vi "2_2_PatchCore_Inference(Camera).vi"() -> ()   [LabVIEW 2020]
uses:
  <vilib>/Ngene/DeepLTK Anomaly Detection Addon/DeepLTK_Anomaly_Detection_Addon/API/Controls/NN_Paths.ctl
  <vilib>/Ngene/Deep Learning Toolkit/Toolkit/NN_Data/API/NN_Dims(C,H,W).ctl
  <vilib>/Ngene/Deep Learning Toolkit/Toolkit/NN_Network/Controls/NN_Device.ctl
  subVIs/Visualizer/Controls/Display_Options.ctl
  subVIs/Visualizer/Controls/ROI_Display_Options.ctl
  subVIs/Visualizer/Controls/Heatmap_Display_Options.ctl
  subVIs/Visualizer/Controls/ColorMap.ctl
  <vilib>/Ngene/DeepLTK Anomaly Detection Addon/DeepLTK_Anomaly_Detection_Addon/API/Controls/MinMax.ctl
  subVIs/Camera/Controls/Camera_Settings.ctl
  <vilib>/vision/driver/IMAQdx.llb/IMAQdx Camera Control Mode.ctl
  <vilib>/Ngene/DeepLTK Anomaly Detection Addon/DeepLTK_Anomaly_Detection_Addon/API/Controls/NNPC_Setup.ctl
  <vilib>/Ngene/DeepLTK Anomaly Detection Addon/DeepLTK_Anomaly_Detection_Addon/API/Controls/Feature_Scorer_Params.ctl
  <vilib>/Ngene/DeepLTK Anomaly Detection Addon/DeepLTK_Anomaly_Detection_Addon/API/Controls/Gaussian_Blur.ctl
  <vilib>/vision/driver/IMAQdx.llb/IMAQdx Buffer Number Mode.ctl
  <vilib>/Ngene/DeepLTK Anomaly Detection Addon/DeepLTK_Anomaly_Detection_Addon/API/NNPC_Predict/NNPC_Predict(Single).vi
  <vilib>/Ngene/DeepLTK Anomaly Detection Addon/DeepLTK_Anomaly_Detection_Addon/DeepLTK_Anomaly_Detection_Addon.lvlib
  <vilib>/ptbypt/NI_PtbyPt.lvlib
  <vilib>/vision/driver/NI_Vision_Acquisition_Software.lvlib
  <vilib>/Ngene/Deep Learning Toolkit/Toolkit/Deep_Learning_Toolkit_by_Ngene.lvlib
  <vilib>/Ngene/CuLab - GPU Accelerated Toolkit/Toolkit/CuLab.lvlib
panel:
  in  "Tab Control":enum32{"CFG", "Demo"}(tab)
  in  "Center_Crop_Size":i32=700
  in  "Device":T1=enum."GPU"
  in  "Trained_Model_Paths":T2={"CFG"=path "D:/working/NI_Connect_PCB/NNPC_PCB5__25_04_11__16_58_48/NNPC_PCB5.cfg", "BIN"=path "D:/working/NI_Connect_PCB/NNPC_PCB5__25_04_11__16_58_48/NNPC_PCB5.bin"}
  in  "Display_Options":T3={"ROI_Options"={"Color"=16711713, "Width"=4, "Drawing Mode"=enum."Frame"}, "Heatmap_Options"={"ColorMap"=enum."Jet", "Alpha"=0.4, "Heatmap Range"={"Min"=38.0, "Max"=-1.0}}, "Has GT?"=FALSE} {"Heatmap_Options"."Heatmap Range"."Min" format="%#_5g"}
  in  "Camera":refnum<k21>="cam3" caption="IMAQdx Session"
  in  "Rel Margin":sgl=0.02
  in  "Camera_Settings":T8={"Camera_Resolution"=39, "Focus"=20, "Exposure"=5, "Gain"=0, "WhiteB."=3000} {"WhiteB." min=2800 max=6500 step=1; "Gain" max=255 step=1; "Exposure" min=0 max=6 step=1; "Focus" step=17}
  out "Loop Time":dbl=0.04018187299996498 format="%.2ps"
  out "Preproc. Time":dbl=0.002760252000152832 format="%.2ps"
  in  "Image_Thrshld":sgl=-1.0 format="%_5g"
  out "Pixel_Score(Max)":sgl=85.97979
  out "Img_Score":sgl=89.875435
  in  "Pixel_Thrshld":sgl=56.0 format="%_5g"
  out "Dims_In":T9={"C"=3, "H"=448, "W"=448}
  in  "Stop":bool
  out "Inference Time":dbl=0.012982828999520279 format="%.2ps"
  out "Prediction":bool=TRUE
  out "Device 2":string="NVIDIA GeForce RTX 2080 Ti"
  out "FPS":dbl=0.012982828999520279 format="%.2ps"
  out "Anomaly Detection Results":T10(plugin-control)
  # "Unsupervised \nVisual Anomaly Detection"
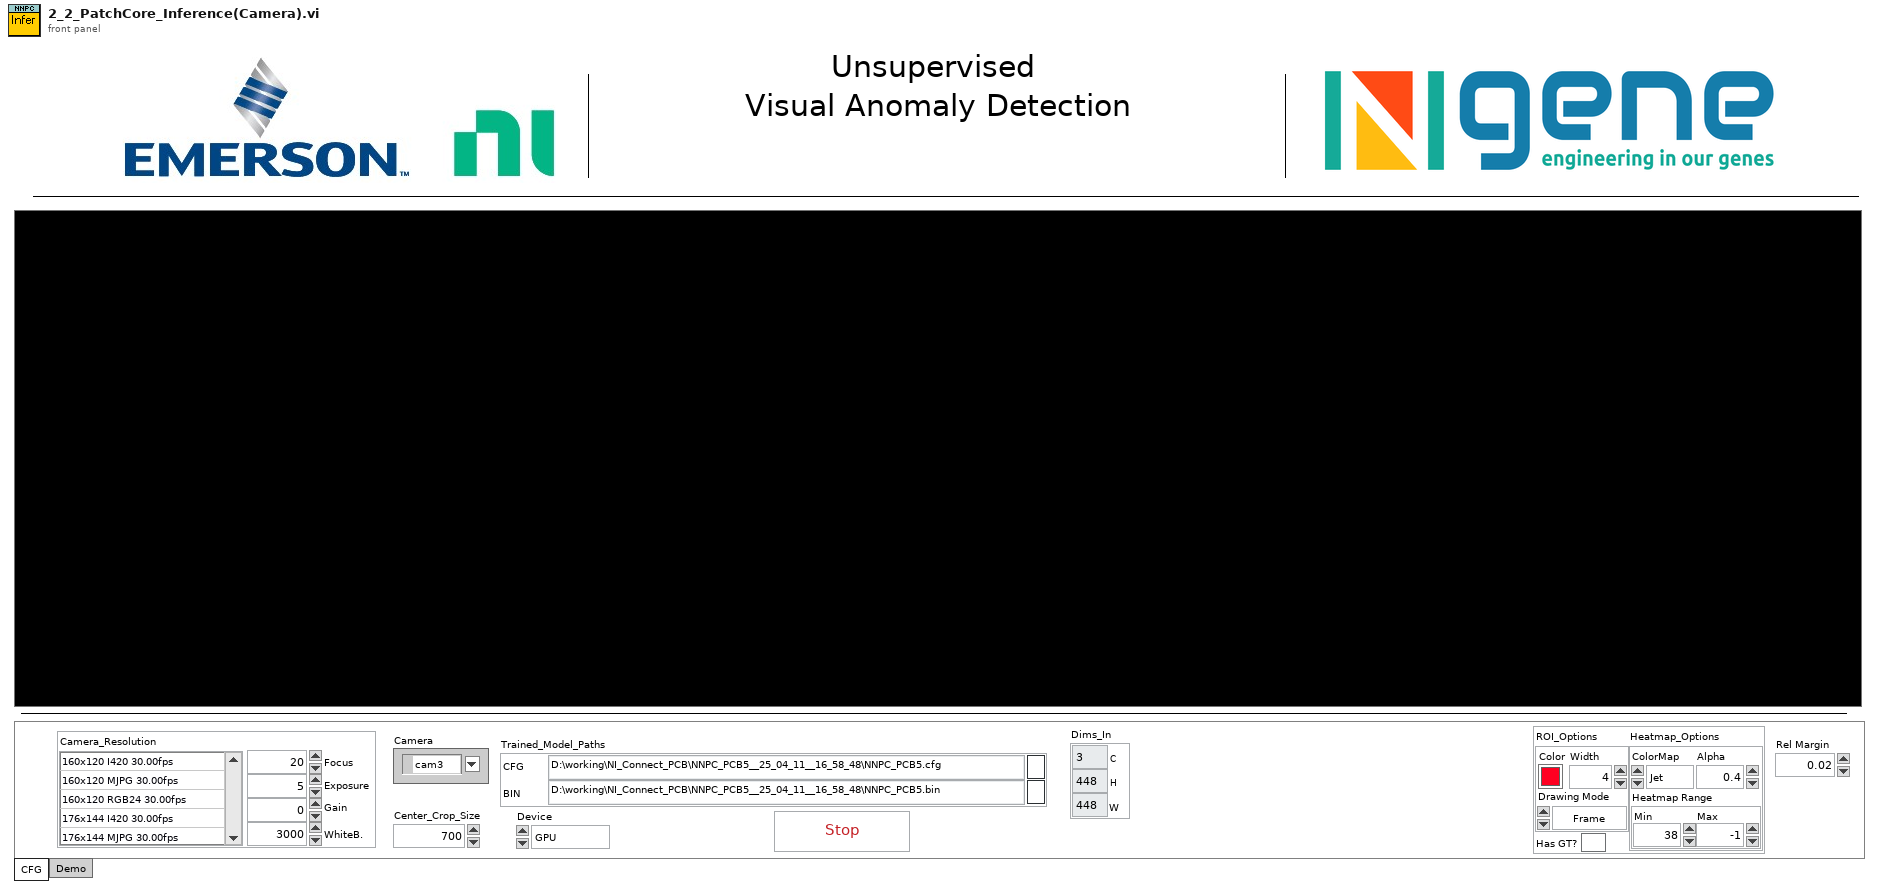
[diagram p1: front panel]
types:
  T1 = typedef "Deep_Learning_Toolkit_by_Ngene.lvlib/NN_Device.ctl" = enum16{"CPU", "GPU"}
  T2 = typedef "DeepLTK_Anomaly_Detection_Addon.lvlib/NN_Paths.ctl" = cluster{"CFG":path, "BIN":path}
  T3 = typedef "Display_Options.ctl" = cluster{"ROI_Options":T4, "Heatmap_Options":T5, "Has GT?":bool}
  T4 = typedef "ROI_Display_Options.ctl" = cluster{"Color":u32, "Width":u32, "Drawing Mode":enum16{"Frame", "Fill"}}
  T5 = typedef "Heatmap_Display_Options.ctl" = cluster{"ColorMap":T6, "Alpha":sgl, "Heatmap Range":T7}
  T6 = typedef "ColorMap.ctl" = enum16{"Jet", "Perula", "Inferno", "Plasma", "Viridis"}
  T7 = typedef "DeepLTK_Anomaly_Detection_Addon.lvlib/MinMax.ctl" = cluster{"Min":sgl, "Max":sgl}
  T8 = typedef "Camera_Settings.ctl" = cluster{"Camera_Resolution":i32, "Focus":u8, "Exposure":i32, "Gain":u32, "WhiteB.":i32}
  T9 = typedef "Deep_Learning_Toolkit_by_Ngene.lvlib/NN_Dims(C,H,W).ctl" = cluster{"C":i32, "H":i32, "W":i32}
  T10 = typedef "IMAQ Image.ctl" = refnum<image>
  T11 = typedef "NI_Vision_Acquisition_Software.lvlib/IMAQdx Camera Control Mode.ctl" = enum32{"Controller", "Listener"}
  T12 = typedef "Image Type" = u32
  T13 = typedef "DeepLTK_Anomaly_Detection_Addon.lvlib/NNPC_Setup.ctl" = cluster{"Input_Dims":T9, "mBatch":i32, "Device":T1, "GPU Id":i32}
  T14 = typedef "IMAQdx.ctl" = refnum<k21>
  T15 = typedef "DeepLTK_Anomaly_Detection_Addon.lvlib/NNPC_Evaluation_Results.ctl" = cluster{"Threshold(Image)":sgl, "Threshold(Pixel)":sgl, "Pixel_Range":cluster{"Min":sgl, "Max":sgl}}
  T16 = typedef "DeepLTK_Anomaly_Detection_Addon.lvlib/NNPC_PreProcessing_Options.ctl" = cluster{"DS_Name":string, "Input_Dims":T9, "Center Crop Size":i32, "Interpolation Type":u32, "Multi-Stage_DownSample?":bool, "Dataset_Stats":T17}
  T17 = typedef "DeepLTK_Anomaly_Detection_Addon.lvlib/NNPC_DS_Stats.ctl" = cluster{"means":T18, "stds":T18}
  T18 = typedef "DeepLTK_Anomaly_Detection_Addon.lvlib/Image_Stats_RGB.ctl" = cluster{"R":sgl, "G":sgl, "B":sgl}
  T19 = typedef "DeepLTK_Anomaly_Detection_Addon.lvlib/NNPC_Instance.ctl" = cluster{"NN":T20, "MemBank_Data":T35, "Name":string}
  T20 = typedef "Deep_Learning_Toolkit_by_Ngene.lvlib/NN.ctl" = cluster{"Name":string, "No of Layers":i32, "mBatch":i32, "Layers":T21[], "Dimty":T22, "Dims_In":T9, "Dims_Out":T9, "Working_Dir":path, "Train?":bool, "Train_Params":T23, "LR_Update_Policy":T26, "Session Data":T28, "Ground_truth":T29, "NNg_hdls":T30, "NN_Device":T1, "GPU Id":i32, "Labels":string[], "Receptive Field":T31[], "Loss_Type":T32, "Loss_Cfg_Prms":variant, "NNG_WS":T33}
  T21 = typedef "Deep_Learning_Toolkit_by_Ngene.lvlib/NN_Layer_ref.ctl" = refnum<data-value>
  T22 = typedef "Deep_Learning_Toolkit_by_Ngene.lvlib/NN_In_Out_Dim-ty.ctl" = enum8{"In1D_Out1D", "In3D_Out1D", "In3D_Out3D", "In3D_OutBBox"}
  T23 = typedef "Deep_Learning_Toolkit_by_Ngene.lvlib/NN_Train_Params.ctl" = cluster{"Optimizer":T24, "Beta_1":sgl, "Beta_2":sgl, "Weight Decay(L1)":sgl, "Weight Decay(L2)":sgl, "Data_Sampling":T25}
  T24 = typedef "Deep_Learning_Toolkit_by_Ngene.lvlib/NN_Train_Optimizer.ctl" = enum16{"SGD", "Adam", "Adagrad", "Adadelta", "RMSProp", "Nesterov"}
  T25 = typedef "Deep_Learning_Toolkit_by_Ngene.lvlib/NN_Train_Data_Sampling.ctl" = enum16{"Random", "Sequential"}
  T26 = typedef "Deep_Learning_Toolkit_by_Ngene.lvlib/NN_LR_Policy_Cfg.ctl" = cluster{"Policy_Type":T27, "LR0":dbl, "k":sgl, "WarmUp_Policy":enum16{"Step", "Ramp"}, "WarmUp_Iter":i32, "WarmUp_Ratio":sgl}
  T27 = typedef "Deep_Learning_Toolkit_by_Ngene.lvlib/NN_LR_Policy_Type.ctl" = enum16{"Manual", "Step", "Exp", "1/t"}
  T28 = typedef "Deep_Learning_Toolkit_by_Ngene.lvlib/NN_Train_Session_Data.ctl" = cluster{"Epochs":sgl, "Tot_Iter":i32, "LR":sgl, "LR_iter":i32}
  T29 = typedef "Deep_Learning_Toolkit_by_Ngene.lvlib/NN_Ground_truth.ctl" = cluster{"Y":variant}
  T30 = typedef "Deep_Learning_Toolkit_by_Ngene.lvlib/nng_cuda_handles.ctl" = cluster{"cudnn":u64, "cublas":u64, "stream":u64, "curand":u64}
  T31 = typedef "Deep_Learning_Toolkit_by_Ngene.lvlib/NN_Dims(V,H).ctl" = cluster{"V":i32, "H":i32}
  T32 = typedef "Deep_Learning_Toolkit_by_Ngene.lvlib/NN_Loss_Type.ctl" = enum16{"None", "MSE", "CrossEntropy", "YOLO_v2", "YOLO_v4"}
  T33 = typedef "Deep_Learning_Toolkit_by_Ngene.lvlib/NNG_WS.ctl" = cluster{"NNG_WS_Mem":T34, "Max_WS_Size":i64}
  T34 = typedef "Deep_Learning_Toolkit_by_Ngene.lvlib/NNg_WS_Mem_DVR.ctl" = refnum<data-value>
  T35 = typedef "DeepLTK_Anomaly_Detection_Addon.lvlib/MemBank_and_Norm_Variants.ctl" = cluster{"MemBank":variant, "MemBank Norm":variant}
  T36 = typedef "DeepLTK_Anomaly_Detection_Addon.lvlib/Feature_Scorer_Params.ctl" = cluster{"Nearest_Neighbors":i32, "Calculate Anomaly Map":bool, "Gaussian_Blur":T37}
  T37 = typedef "DeepLTK_Anomaly_Detection_Addon.lvlib/Gaussian_Blur.ctl" = cluster{"Kernel_Size":i32, "Sigma":sgl}
  T38 = typedef "NI_Vision_Acquisition_Software.lvlib/IMAQdx Buffer Number Mode.ctl" = enum32{"Next", "Last", "Buffer Number", "Every", "Last New"}
  T39 = typedef "Anomaly_Detection_Results_Imgs.ctl" = cluster{"Image":T10, "Ground Truth":T10, "Predicted Heat Map":T10, "Predicted Mask":T10, "Segmentation":T10}
  T40 = typedef "CuLab.lvlib/Properties.ctl" = cluster{"Device ID":i32, "Name":string}
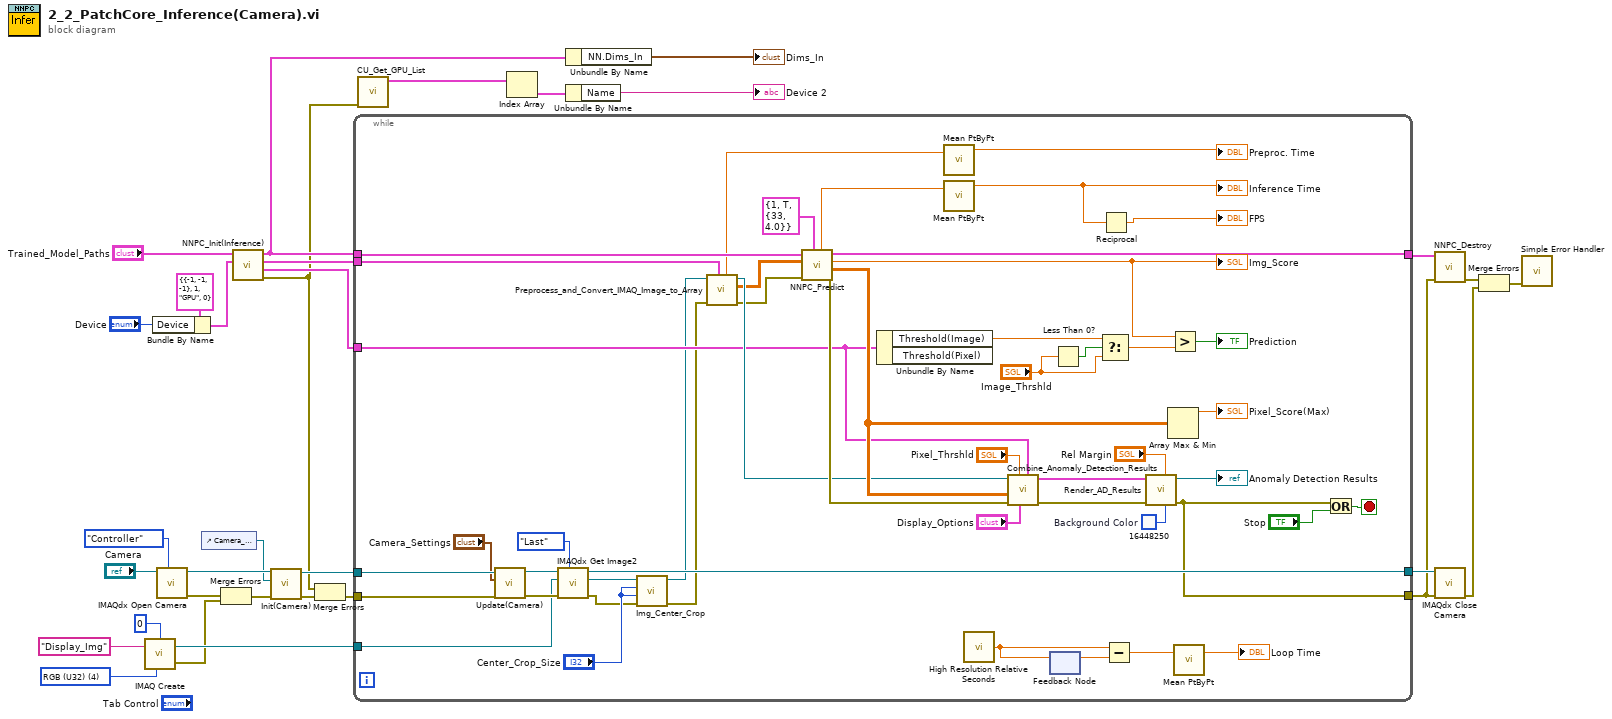
[diagram p0: block diagram]
diagram:
  w12 = T12 4 items=["Grayscale (U8)", "Grayscale (I16)", "Grayscale (SGL)", "Complex (CSG)", "RGB (U32)", "HSL (U32)", "RGB (U64)", "Grayscale (U16)"] ("Image Type")
  n1 = call "IMAQ Create"("Border Size"=0, "Image Name"="Display_Img", "Image Type"=w12) -> ("New Image"=w6:T10, "error out"=w3:errorcluster)  [unwired: 2 in]
  n2 = Bundle By Name(cluster=T13 {"Input_Dims"={"C"=-1, "H"=-1, "W"=-1}, "mBatch"=1, "Device"=enum."GPU", "GPU Id"=0} ("NNFE_CFG"), "Device"="Device") -> (w5:T13)
  n3 = call <vilib>:"IMAQdx Open Camera.vi"("Camera Control Mode"=IMAQdx_Camera_Control_Mode."Controller", "Session In"="Camera") -> ("error out"=w13:errorcluster, "Session Out"=w14:T14)  [unwired: 1 in, 7 out]
  n4 = control-ref of="Camera_Settings"() -> (w4:refnum<vi>)
  n5 = Merge Errors(w13, w3) -> (w9:errorcluster)
  n6 = call <vilib>:"NNPC_Init(Inference).vi"("NNPC_Setup"=w5, "NNPC_Paths"="Trained_Model_Paths") -> ("error out"=w1:errorcluster, "Evaluation_Results"=w28:T15, "PreProc_Options"=w29:T16, "NNPC_out"=w23:T19)  [unwired: 5 in, 1 out]
  n7 = call "Init(Camera).vi"("error in (no error)"=w9, "Camera_Settings_Ref"=w4, "Session in"=w14) -> ("error out"=w8:errorcluster, "Session out"=w7:T14)  [unwired: 7 in]
  n8 = Merge Errors(w1, w8) -> (w2:errorcluster)
  n9 = while {
    tunnel: w23 -> [w71]
    tunnel: [w66] -> w32
    tunnel: w29 -> [w56]
    tunnel: w28 -> [w51]
    tunnel: [w58] -> w27
    tunnel: [w50] -> w24
    tunnel: w2 -> [w42]
    tunnel: w7 -> [w45]
    tunnel: w6 -> [w41]
    stop <- w65 stop-if-true
    w64 = u32 16448250  # Background Color
    n10 = call "Update(Camera).vi"("error in (no error)"=w42, "Camera_Settings"="Camera_Settings", "Session in"=w45) -> ("error out"=w44:errorcluster, "Session out"=w43:T14)  [unwired: 7 in]
    n11 = call <vilib>:"IMAQdx Get Image2.vi"("Buffer Number Mode (Next)"=IMAQdx_Buffer_Number_Mode."Last", "error in"=w44, "Image In"=w41, "Session In"=w43) -> ("error out"=w37:errorcluster, "Image Out"=w57:T10, "Session Out"=w58:T14)  [unwired: 4 in, 1 out]
    n12 = call "Img_Center_Crop.vi"("error in (no error)"=w37, "height"="Center_Crop_Size", "width"="Center_Crop_Size", "Image In"=w57) -> ("error out"=w36:errorcluster, "Image Out"=w39:T10)  [unwired: 6 in]
    n13 = call "Preprocess_and_Convert_IMAQ_Image_to_Array.vi"("PreProcessing_Options"=w56, "error in (no error)"=w36, "Imaq Image In"=w39) -> ("error out"=w52:errorcluster, "Norm_Img_Out"=w35:sgl[][][], "Imaq Image Out"=w53:T10, "dT_Preprocessing"=w54:dbl)  [unwired: 5 in]
    n14 = call-poly <vilib>:"NNPC_Predict.vi"("Feature_Scorer_Params"=T36 {"Nearest_Neighbors"=1, "Calculate Anomaly Map"=TRUE, "Gaussian_Blur"={"Kernel_Size"=33, "Sigma"=4.0}}, "error in"=w52, "Image_in"=w35, "NNPC_in"=w71) -> ("error out"=w81:errorcluster, "Anomaly_Map"=w70:sgl[][], "Pred_Score"=w69:sgl, "NNPC_out"=w66:T19, "dT_Predict"=w63:dbl)  [unwired: 3 in]
    "Img_Score" <- w69
    n15 = Unbundle By Name(w51) -> ("Threshold(Image)"=w62:sgl)  [unwired: 1 out]
    n16 = call <vilib>:"Mean PtByPt.vi"("x"=w54) -> ("mean"=→"Preproc. Time":dbl)  [unwired: 3 in, 1 out]
    n17 = call <vilib>:"Mean PtByPt.vi"("x"=w63) -> ("mean"=w34:dbl)  [unwired: 3 in, 1 out]
    "Inference Time" <- w34
    n18 = call <vilib>:"High Resolution Relative Seconds.vi"() -> ("relative seconds"=w60:dbl)
    n19 = call "Combine_Anomaly_Detection_Results.vi"("Evaluation_Results"=w51, "Display_Options"="Display_Options", "Pixel Anomaly Thrshld"="Pixel_Thrshld", "error in"=w81, "Anomaly Map"=w70, "Orig Image In"=w53) -> ("error out"=w80:errorcluster, "Anomaly Detection Rresults"=w79:T39)  [unwired: 3 in, 1 out]
    n20 = feedback #1() -> (w61:dbl)  [unwired: 1 in]
    n21 = feedback-in #1(w60) -> ()
    n22 = Less Than 0?(x="Image_Thrshld") -> (x < 0?=w75:bool)
    n23 = Select(t=w62, s=w75, f="Image_Thrshld") -> (s? t:f=w73:sgl)
    n24 = Reciprocal(x=w34) -> (1/x=→"FPS":dbl)
    n25 = Subtract(x=w60, y=w61) -> (x-y=w59:dbl)
    n26 = call "Render_AD_Results.vi"("Background Color"=w64, "Rel._Margin"="Rel Margin", "error in"=w80, "Anomaly Detection Rresults"=w79) -> ("error out"=w50:errorcluster, "Anomaly Detection Results"=→"Anomaly Detection Results":T10)  [unwired: 6 in]
    n27 = Array Max & Min(array=w70) -> (max value=→"Pixel_Score(Max)":sgl)  [unwired: 3 out]
    n28 = Greater?(x=w69, y=w73) -> (0:→"Prediction":bool)
    n29 = call <vilib>:"Mean PtByPt.vi"("x"=w59) -> ("mean"=→"Loop Time":dbl)  [unwired: 3 in, 1 out]
    n30 = Or(x=w50, y="Stop") -> (x .or. y?=w65:bool)
  }
  n31 = call <vilib>:"CU_Get_GPU_List.vi"("error in (no error)"=w1) -> ("Devices"=w19:T40[])  [unwired: 9 in, 1 out]
  n32 = Index Array(array=w19) -> (element=w18:T40)  [unwired: 1 in]
  n33 = Unbundle By Name(w23) -> ("NN.Dims_In"=→"Dims_In":T9)
  n34 = Unbundle By Name(w18) -> ("Name"=→"Device 2":string)
  n35 = call <vilib>:"NNPC_Destroy.vi"("error in"=w24, "NNPC_in"=w32) -> ("error out"=w31:errorcluster)  [unwired: 9 in]
  n36 = call <vilib>:"IMAQdx Close Camera.vi"("error in"=w24, "Session In"=w27) -> ("error out"=w25:errorcluster)  [unwired: 9 out]
  n37 = Merge Errors(w31, w25) -> (w26:errorcluster)
  n38 = call <vilib>:"Simple Error Handler.vi"("error in (no error)"=w26) -> ()  [unwired: 4 in, 5 out]
